vi "MindwaveAUTO.vi"(3 "error in (no error) input":errorcluster, 5 "VISA resource name input":refnum<visa-resource-name>) -> (0 "error out":errorcluster, 1 "MindWave":T1, 2 "VISA resource name out":refnum<visa-resource-name>)   [LabVIEW 2011, in "Neurosky.lvlib"]
uses:
  Users/Isaias/Documents/GitHub/Neurosky/Neurosky.lvlib
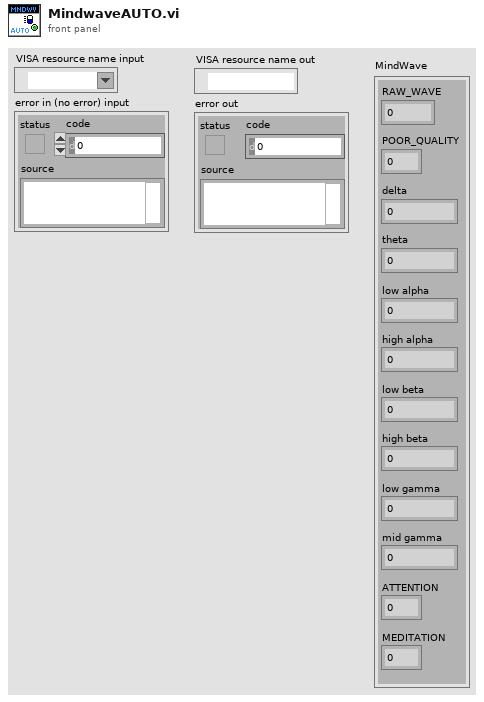
[diagram p1: front panel]
types:
  T1 = cluster{"RAW_WAVE":i16, "POOR_QUALITY":u8, "delta":sgl, "theta":sgl, "low alpha":sgl, "high alpha":sgl, "low beta":sgl, "high beta":sgl, "low gamma":sgl, "mid gamma":sgl, "ATTENTION":u8, "MEDITATION":u8}
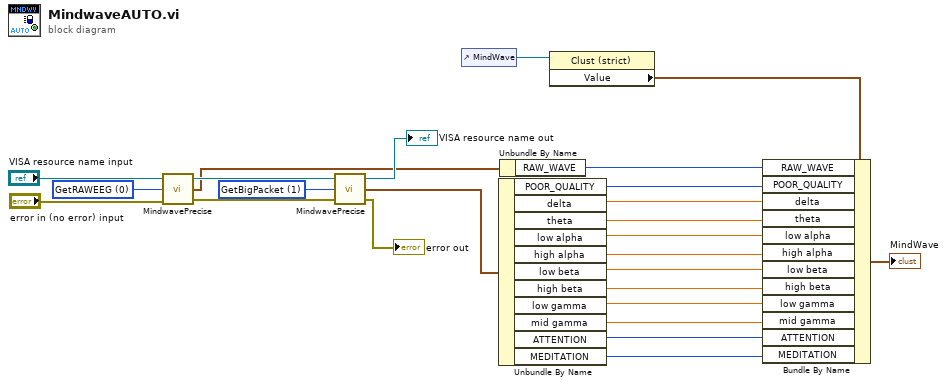
[diagram p0: block diagram]
diagram:
  w24 = u16 1 items=["GetRAWEEG", "GetBigPacket"] ("Control Box")
  w25 = u16 0 items=["GetRAWEEG", "GetBigPacket"] ("Control Box")
  n1 = call <userlib>:"MindwavePrecise.vi"("error in (no error) input"="error in (no error) input", "Control Box"=w25, "VISA resource name input"="VISA resource name input") -> ("error out"=w9:errorcluster, "MindWave"=w5:T1, "VISA resource name out"=w10:refnum<visa-resource-name>)
  n2 = call <userlib>:"MindwavePrecise.vi"("error in (no error) input"=w9, "Control Box"=w24, "VISA resource name input"=w10) -> ("error out"=→"error out":errorcluster, "MindWave"=w4:T1, "VISA resource name out"=→"VISA resource name out":refnum<visa-resource-name>)
  n3 = control-ref of="MindWave"() -> (w2:refnum<vi>)
  n4 = Unbundle By Name(w4) -> ("POOR_QUALITY"=w23:u8, "delta"=w13:sgl, "theta"=w14:sgl, "low alpha"=w15:sgl, "high alpha"=w16:sgl, "low beta"=w17:sgl, "high beta"=w18:sgl, "low gamma"=w19:sgl, "mid gamma"=w20:sgl, "ATTENTION"=w21:u8, "MEDITATION"=w22:u8)
  n5 = Unbundle By Name(w5) -> ("RAW_WAVE"=w6:i16)
  n6 = property on="Property Node" class="Clust (strict)"(reference=w2) -> ("Value"=w3:T1)  [unwired: 1 in, 2 out]
  n7 = Bundle By Name(cluster=w3, "RAW_WAVE"=w6, "POOR_QUALITY"=w23, "delta"=w13, "theta"=w14, "low alpha"=w15, "high alpha"=w16, "low beta"=w17, "high beta"=w18, "low gamma"=w19, "mid gamma"=w20, "ATTENTION"=w21, "MEDITATION"=w22) -> (→"MindWave":T1)
